vi "Start Acquisition.vi"(8 "error in (no error)":errorcluster, 11 "CCDCamera in":refnum<class "CCDCamera.lvclass">) -> (0 "error out":errorcluster, 3 "CCDCamera out":refnum<class "CCDCamera.lvclass">)   [LabVIEW 2018, in "CCDCamera.lvclass"]
uses:
  CCDCamera.lvclass
  CCDCamera.lvclass/CCDCamera.ctl
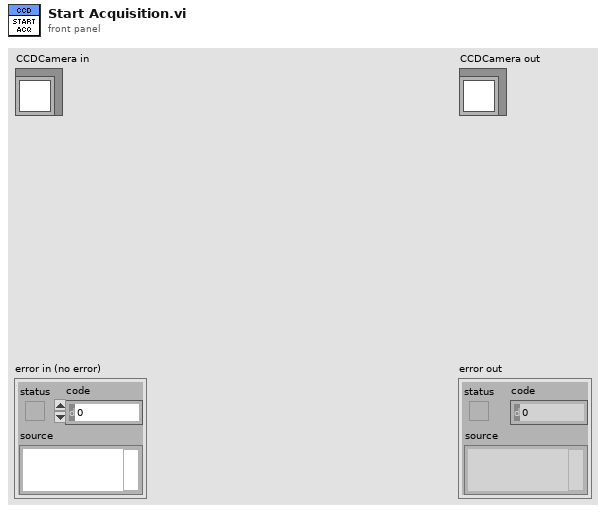
[diagram p1: front panel]
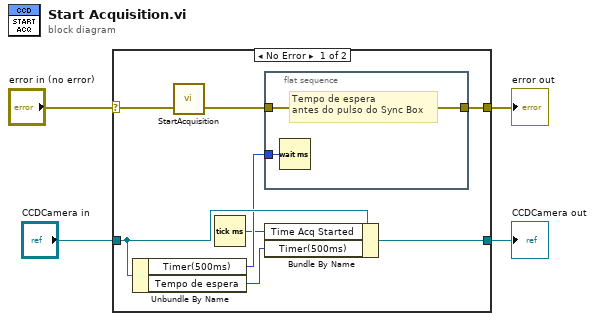
[diagram p0: block diagram]
diagram:
  n1 = case shown="No Error" "error in (no error)" {
    selector: "error in (no error)" -> [w12 w16]
    tunnel: [w8 w16] -> w3
    tunnel: [w10 w15] -> w1
    tunnel: "CCDCamera in" -> [w11 w15]
    frame No Error {
      n2 = Unbundle By Name(w11) -> ("Timer(500ms)"=w7:u16, "Tempo de espera"=w6:u16)
      n3 = call <userlib>:"StartAcquisition.vi"("error in (no error)"=w12) -> ("error out"=w9:errorcluster)  [unwired: 1 in, 1 out]
      n4 = Tick Count (ms)() -> (millisecond timer value=w5:u32)
      n5 = flat-sequence {
        tunnel: w9 -> [w14]
        tunnel: w7 -> [w13]
        tunnel: [w14] -> w8
        frame #0 {
          # "Tempo de espera\nantes do pulso do Sync Box"
          n6 = Wait (ms)(milliseconds to wait=w13) -> ()  [unwired: 1 out]
        }
      }
      n7 = Bundle By Name(cluster=w11, "Time Acq Started"=w5, "Timer(500ms)"=w6) -> (w10:refnum<class "CCDCamera.lvclass">)
    }
    frame Error {
    }
  }
  "error out" <- w3
  "CCDCamera out" <- w1
